vi "Decimation.vi"(8 "error in (no error)":errorcluster, 11 "Node Ptr":T1 format="%.0x") -> (0 "error out":errorcluster)   [LabVIEW 2026, in "Nominal Core Streaming System Explorer.lvlib"]
uses:
  Nominal Core Streaming System Explorer.lvlib
  <vilib>/NI VeriStand/Custom Device API/Custom Device Item Ref.ctl
  <vilib>/NI VeriStand/Custom Device API/Custom Device API.lvlib
panel:
  in  "initial decimation":u32=1 min=1 step=1
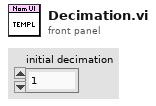
[diagram p1: front panel]
types:
  T1 = typedef "Custom Device API.lvlib/Custom Device Item Ref.ctl" = u64
  T2 = typedef "Custom Device API.lvlib/Custom Device Channel.ctl" = cluster{"Type":T3, "Units":string, "Default Value":dbl, "Faultable":bool, "Scalable":bool}
  T3 = typedef "Custom Device API.lvlib/Custom Device Channel Type.ctl" = enum16{"Input", "Output"}
  T4 = typedef "Custom Device API.lvlib/Custom Device Commands.ctl" = enum16{"Default", "Item renamed", "Shutdown", "Dynamic button pressed"}
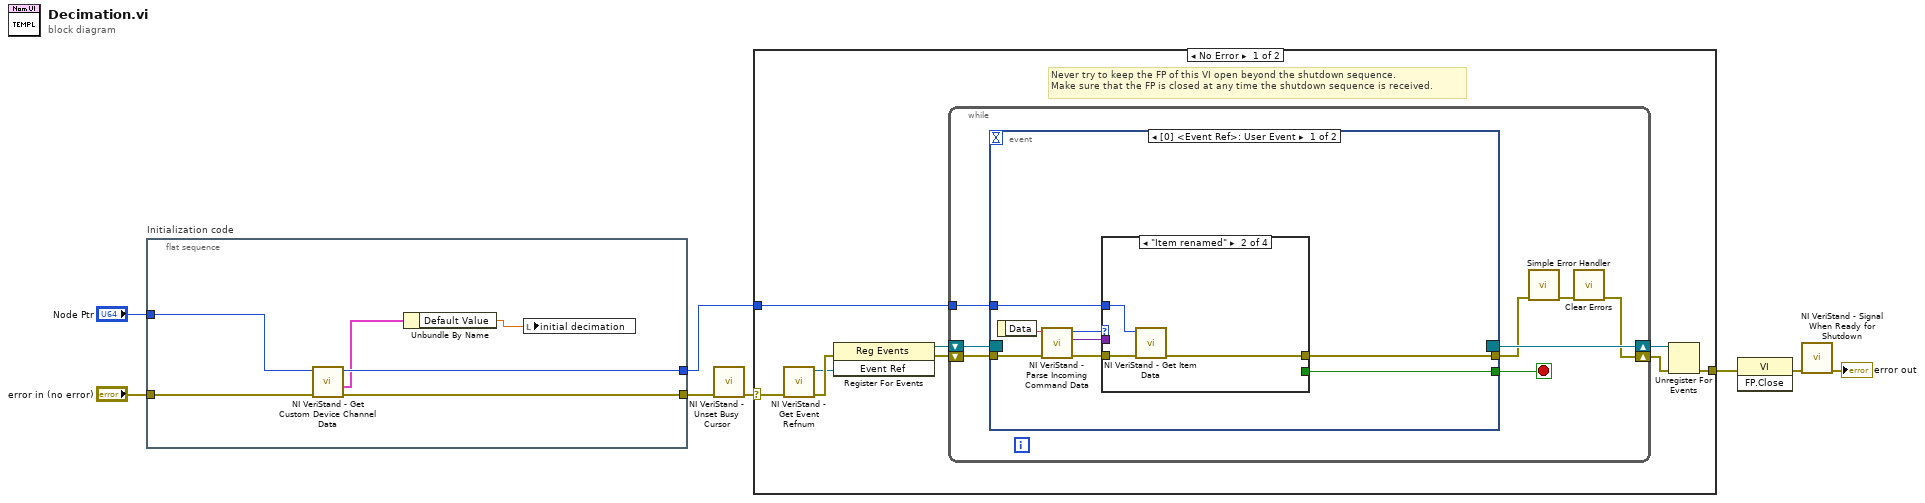
[diagram p0: block diagram]
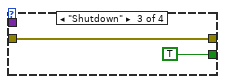
[diagram p3: hidden frame]
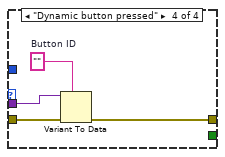
[diagram p4: hidden frame]
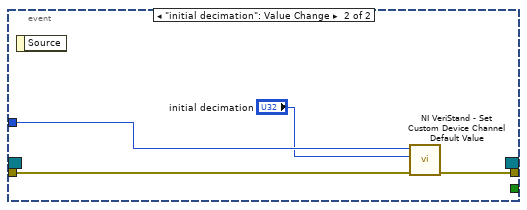
[diagram p5: hidden frame]
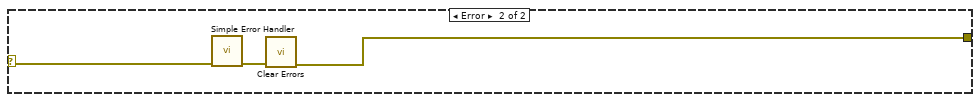
[diagram p6: hidden frame]
diagram:
  n1 = flat-sequence "Initialization code" {
    tunnel: "error in (no error)" -> [w14]
    tunnel: "Node Ptr" -> [w12]
    tunnel: [w13] -> w4
    tunnel: [w11] -> w1
    frame #0 {
      n2 = call <vilib>:"NI VeriStand - Get Custom Device Channel Data.vi"("error in (no error)"=w14, "Channel Ref in"=w12) -> ("error out"=w13:errorcluster, "Channel"=w10:T2, "Channel Ref out"=w11:T1)  [unwired: 4 in, 3 out]
      n3 = Unbundle By Name(w10) -> ("Default Value"=w9:dbl)
      n4 = local write "initial decimation"(w9) -> ()
    }
  }
  n5 = call <vilib>:"NI VeriStand - Unset Busy Cursor.vi"("error in (no error)"=w4) -> ("error out"=w3:errorcluster)  [unwired: 10 out]
  n6 = case shown="No Error" w3 {
    selector: w3 -> [w15 w56]
    tunnel: [w20 w54] -> w8
    tunnel: w1 -> [w16 _]
    frame No Error {
      # "Never try to keep the FP of this VI open beyond the shutdown sequence.\nMake sure that the FP is closed at any time the shutdown sequence is received."
      n7 = call <vilib>:"NI VeriStand - Get Event Refnum.vi"("error in (no error)"=w15) -> ("error out"=w23:errorcluster, "Event Ref"=w19:refnum<user-event>)  [unwired: 9 out]
      n8 = register-events(error in=w23, w19) -> (reference out=w17:refnum<event-registration>, error out=w18:errorcluster)  [unwired: 1 in]
      n9 = while {
        tunnel: w16 -> [w27]
        shift-right: [w24] -> w21
        shift-left: w18 -> [w30]
        shift-right: [w31] -> w22
        shift-left: w17 -> [w29]
        stop <- w28 stop-if-true
        n10 = event shown="[0] <Event Ref>: User Event" {
          selector: w29 -> [_ _]
          dyn-events: [_ _] -> w31
          timeout: _ -> [_ _]
          tunnel: w30 -> [w39 w53]
          tunnel: [w35 _] -> w28
          tunnel: [w34 w52] -> w26
          tunnel: w27 -> [w33 w51]
          event User Event {
            n11 = event-data() -> ("Data"=w38:string)  [unwired: 1 out]
            n12 = call <vilib>:"NI VeriStand - Parse Incoming Command Data.vi"("error in (no error)"=w39, "Incoming data"=w38) -> ("error out"=w37:errorcluster, "Outgoing data"=w32:variant, "Action"=w36:T4)  [unwired: 7 out]
            n13 = case shown="\"Item renamed\"" w36 {
              tunnel: w37 -> [w40 w43 w44 w49]
              tunnel: [_ _ TRUE _] -> w35
              tunnel: [w40 w41 w44 w46] -> w34
              tunnel: w33 -> [_ w42 _ _]
              tunnel: w32 -> [_ _ _ w48]
              frame "Default", Default {
              }
              frame "Item renamed" {
                n14 = call <vilib>:"NI VeriStand - Get Item Data.vi"("error in (no error)"=w43, "Item Ref in"=w42) -> ("error out"=w41:errorcluster)  [unwired: 9 out]
              }
              frame "Shutdown" {
              }
              frame "Dynamic button pressed" {
                w47 = ""  # Button ID
                n15 = Variant To Data(error in=w49, type=w47, Variant=w48) -> (error out=w46:errorcluster)  [unwired: 1 out]
              }
            }
          }
          event "initial decimation": Value Change {
            n16 = event-data() -> ()  [unwired: 2 out]
            n17 = call <vilib>:"NI VeriStand - Set Custom Device Channel Default Value.vi"("error in (no error)"=w53, "Default Value"="initial decimation", "Channel Ref in"=w51) -> ("error out"=w52:errorcluster)  [unwired: 7 in, 1 out]
          }
        }
        n18 = call <vilib>:"Simple Error Handler.vi"("error in (no error)"=w26) -> ("error out"=w25:errorcluster)  [unwired: 1 in, 7 out]
        n19 = call <vilib>:"Clear Errors.vi"("error in (no error)"=w25) -> ("error out"=w24:errorcluster)  [unwired: 1 in, 5 out]
      }
      n20 = Unregister For Events(event registration refnum=w22, error in=w21) -> (error out=w20:errorcluster)
    }
    frame Error {
      n21 = call <vilib>:"Simple Error Handler.vi"("error in (no error)"=w56) -> ("error out"=w55:errorcluster)  [unwired: 1 in, 7 out]
      n22 = call <vilib>:"Clear Errors.vi"("error in (no error)"=w55) -> ("error out"=w54:errorcluster)  [unwired: 1 in, 5 out]
    }
  }
  n23 = invoke class="VI" method="FP.Close"(error in=w8) -> (error out=w7:errorcluster)  [unwired: 2 in, 2 out]
  n24 = call <vilib>:"NI VeriStand - Signal When Ready for Shutdown.vi"("error in (no error)"=w7) -> ("error out"=→"error out":errorcluster)  [unwired: 10 out]
